vi "3D Scanner - Scanbeweging  - LASER MOVEMENT.vi"() -> ()   [LabVIEW 2012]
uses:
  <vilib>/Instr/_visa.llb/VISA Configure Serial Port (Instr).vi
panel:
  in  "Select COM Port 2":refnum<visa-resource-name>="COM4"
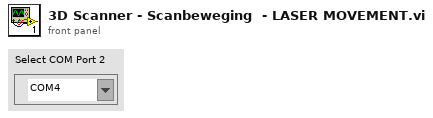
[diagram p1: front panel]
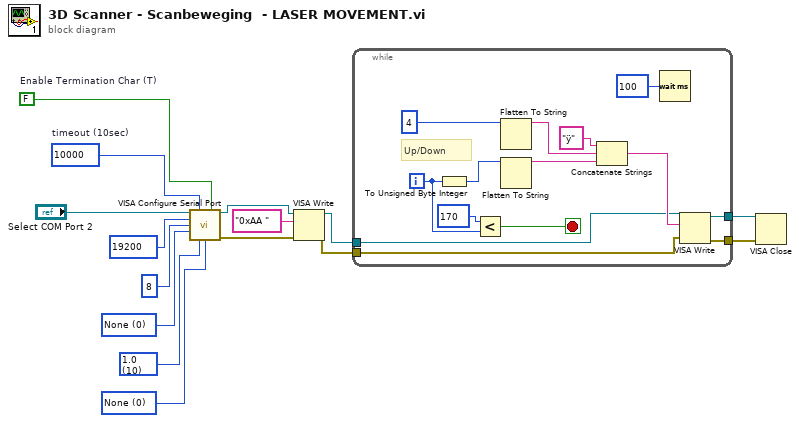
[diagram p0: block diagram]
diagram:
  w13 = u16 0 items=["None"=0, "XON/XOFF"=1, "RTS/CTS"=2, "DTR/DSR"=4] ("flow control")
  w12 = u16 10 items=["1.0"=10, "1.5"=15, "2.0"=20] ("stop bits")
  w11 = u16 0 items=["None", "Odd", "Even", "Mark", "Space"] ("parity")
  w8 = FALSE  # Enable Termination Char (T)
  w7 = u32 10000  # timeout (10sec)
  n1 = call-poly "VISA Configure Serial Port"("VISA resource name"="Select COM Port 2", "timeout (10sec)"=w7, "Enable Termination\nChar (T)"=w8, "baud rate (9600)"=u32 19200 ("baud rate"), "data bits (8)"=u16 8 ("data bits"), "parity (0:none)"=w11, "stop bits (10: 1 bit)"=w12, "flow control (0:none)"=w13) -> ("VISA resource name out"=w15:refnum<visa-resource-name>, "error out"=w14:errorcluster)  [unwired: 1 in, 5 out]
  n2 = VISA Write(VISA resource name=w15, write buffer="0xAA ", error in (no error)=w14) -> (VISA resource name out=w4:refnum<visa-resource-name>, error out=w3:errorcluster)  [unwired: 1 out]
  n3 = while {
    tunnel: [w22] -> w2
    tunnel: [w21] -> w1
    tunnel: w4 -> [w17]
    tunnel: w3 -> [w16]
    i -> [w19]
    stop <- w29 stop-if-true
    # "Up/Down"
    n4 = To Unsigned Byte Integer(number=w19) -> (unsigned 8bit integer=w20:u8)
    n5 = Less?(x=170, y=w19) -> (x < y?=w29:bool)
    n6 = Flatten To String(anything=u8 4) -> (data string=w25:string)  [unwired: 1 in, 4 out]
    n7 = Flatten To String(anything=w20) -> (data string=w26:string)  [unwired: 2 in, 3 out]
    n8 = Concatenate Strings("ÿ", w25, w26) -> (w23:string)
    n9 = Wait (ms)(milliseconds to wait=u32 100) -> ()  [unwired: 1 out]
    n10 = VISA Write(VISA resource name=w17, write buffer=w23, error in (no error)=w16) -> (VISA resource name out=w22:refnum<visa-resource-name>, error out=w21:errorcluster)  [unwired: 1 out]
  }
  n11 = VISA Close(VISA resource name=w2, error in (no error)=w1) -> ()  [unwired: 1 out]
